vi "Set Title.vi"(10 "Title":string) -> ()   [LabVIEW 2014, in "Endigit.lvlib"]
uses:
  Endigit.lvlib
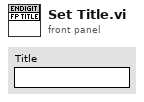
[diagram p1: front panel]
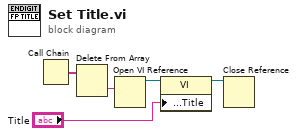
[diagram p0: block diagram]
diagram:
  n1 = Call Chain() -> (call chain=w4:string[])
  n2 = Delete From Array(array=w4) -> (deleted portion=w3:string)  [unwired: 2 in, 1 out]
  n3 = Open VI Reference(vi path=w3) -> (vi reference=w2:refnum<vi>)  [unwired: 5 in, 1 out]
  n4 = property class="VI"(reference=w2, "Front Panel Window:Title"="Title") -> (reference out=w1:refnum<vi>)  [unwired: 1 in, 1 out]
  n5 = Close Reference(reference=w1) -> ()  [unwired: 1 in, 1 out]
